vi "read_attributes.vi"(8 "error in (no error)":errorcluster, 11 "MiniBatchSparsePCA in":refnum<class "MiniBatchSparsePCA.lvclass">) -> (0 "error out":errorcluster, 2 "attributes":T1, 3 "MiniBatchSparsePCA out":refnum<class "MiniBatchSparsePCA.lvclass">)   [LabVIEW 2020, in "MiniBatchSparsePCA.lvclass"]
uses:
  MiniBatchSparsePCA.lvclass
  Controls/mini_batch_sparse_pca_attributes.ctl
  MiniBatchSparsePCA.lvclass/MiniBatchSparsePCA.ctl
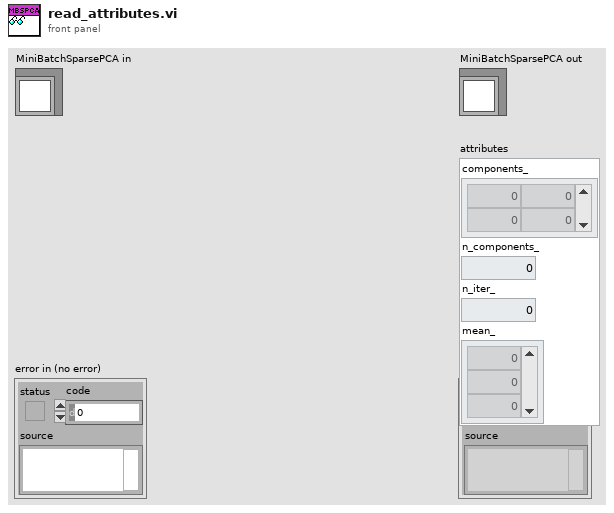
[diagram p1: front panel]
types:
  T1 = typedef "mini_batch_sparse_pca_attributes.ctl" = cluster{"components_":dbl[][], "n_components_":dbl, "n_iter_":dbl, "mean_":dbl[]}
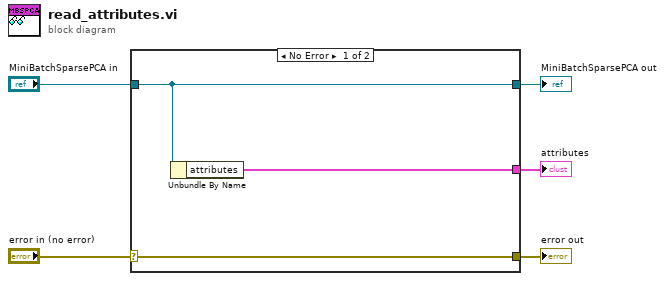
[diagram p0: block diagram]
diagram:
  n1 = case shown="No Error" "error in (no error)" {
    selector: "error in (no error)" -> [w8 w9]
    tunnel: [w8 w9] -> w4
    tunnel: [w7 w10] -> w2
    tunnel: "MiniBatchSparsePCA in" -> [w7 w10]
    tunnel: [w6 _] -> w1
    frame No Error {
      n2 = Unbundle By Name(w7) -> ("attributes"=w6:T1)
    }
    frame Error {
    }
  }
  "error out" <- w4
  "MiniBatchSparsePCA out" <- w2
  "attributes" <- w1
